vi "Git_Demo.vi"() -> ()   [LabVIEW 2015]
panel:
  out "x+y":dbl
  in  "숫자형 2":dbl
  in  "숫자형":dbl
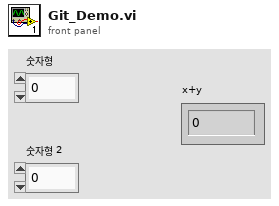
[diagram p1: front panel]
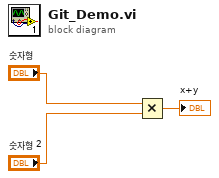
[diagram p0: block diagram]
diagram:
  n1 = Multiply(x="숫자형", y="숫자형 2") -> (x*y=→"x+y":dbl)
